vi "20170502-lecture4-1 read data from file txt.vi"() -> ()   [LabVIEW 2014]
panel:
  out "Array":dbl[](array[numeric])
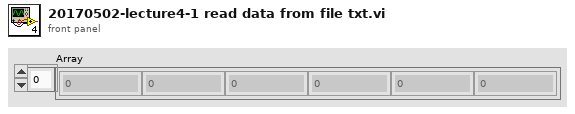
[diagram p1: front panel]
types:
  T1 = enum16{"open", "replace", "create", "open or create", "replace or create", "replace or create with confirmation"}
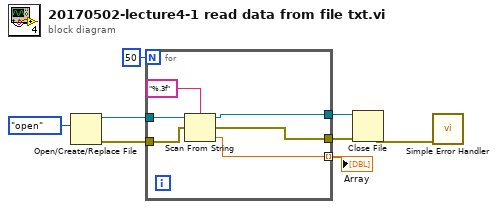
[diagram p0: block diagram]
diagram:
  n1 = Open/Create/Replace File(operation (0:open)=T1."open") -> (refnum out=w6:refnum<file>, error out=w5:errorcluster)  [unwired: 5 in, 1 out]
  n2 = for {
    N: 50 -> [_]
    tunnel: w6 -> [w14]
    tunnel: w5 -> [w13]
    tunnel: [w12] -> w1 mode=indexing
    tunnel: [w11] -> w4
    tunnel: [w10] -> w3
    n3 = Scan From String("%.3f" ("format string"), w14, w13) -> (w11:refnum<file>, w10:errorcluster, output 1=w12:dbl)  [unwired: 1 in]
  }
  "Array" <- w1
  n4 = Close File(refnum=w4, error in=w3) -> (error out=w2:errorcluster)  [unwired: 1 out]
  n5 = call <vilib>:"Simple Error Handler.vi"("error in (no error)"=w2) -> ()  [unwired: 4 in, 5 out]
